vi "GetTunnels.vi"(6 "error in":errorcluster, 9 "Loop in":refnum<class "Loop.lvclass">) -> (0 "error out":errorcluster, 3 "Loop out":refnum<class "Loop.lvclass">, 4 "Tunnels":i32[](array[numeric]))   [LabVIEW 2014]
uses:
  Loop.lvclass
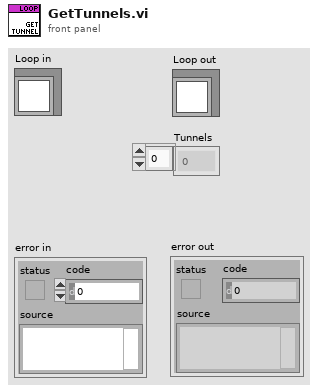
[diagram p1: front panel]
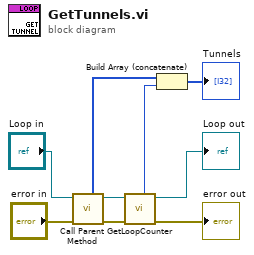
[diagram p0: block diagram]
diagram:
  n1 = call-parent "Call Parent Method"("error in"="error in", "Structure in"="Loop in") -> ("error out"=w6:errorcluster, "Structure out"=w7:refnum<class "Loop.lvclass">, "Tunnels"=w3:i32[])  [unwired: 5 in]
  n2 = call "GetLoopCounter.vi"("error in"=w6, "Loop in"=w7) -> ("error out"=→"error out":errorcluster, "Loop out"=→"Loop out":refnum<class "Loop.lvclass">, "counter UID"=w2:i32)  [unwired: 5 in]
  n3 = Build Array (concatenate)(w3, w2) -> (→"Tunnels":i32[])
